vi "Read DIP Switches.vi"(8 "error in":errorcluster, 10 "Amount of Switches":i32=3, 11 "HBDeviceRef In":T1) -> (0 "error out":errorcluster, 1 "Boolean Array":bool[](array[boolean]), 2 "Index":dbl, 3 "HBDeviceRef Out":T1)   [LabVIEW 2016]
uses:
  <vilib>/Rock Robotics/WPI/SerialPort/WPI_SerialPortRef.ctl
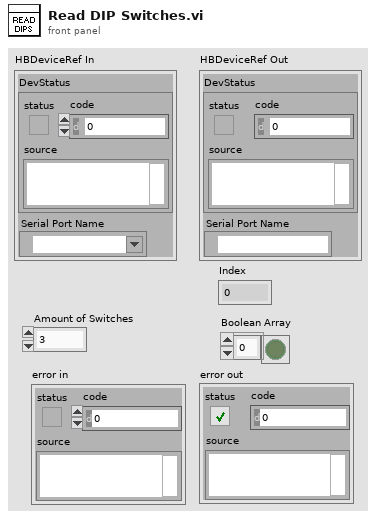
[diagram p1: front panel]
types:
  T1 = typedef "WPI_SerialPortRef.ctl" = cluster{"DevStatus":errorcluster, "Serial Port Name":refnum<visa-resource-name>}
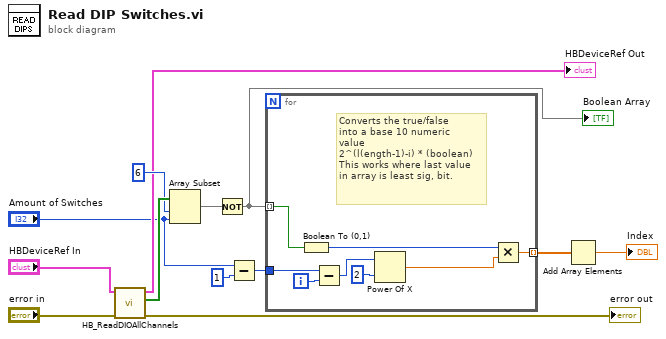
[diagram p0: block diagram]
diagram:
  n1 = call <vilib>:"HB_ReadDIOAllChannels.vi"("error in (no error)"="error in", "HBDeviceRef"="HBDeviceRef In") -> ("error out"=→"error out":errorcluster, "All Digital Input Vals"=w12:bool[], "HBDeviceRef"=→"HBDeviceRef Out":T1)  [unwired: 7 in]
  n2 = Array Subset(array=w12, index=6, length="Amount of Switches") -> (w10:bool[])
  n3 = Not(x=w10) -> (.not. x?=w9:bool[])
  "Boolean Array" <- w9
  n4 = Subtract(x="Amount of Switches", y=1) -> (x-y=w1:i32)
  n5 = for {
    tunnel: w9 -> [w16] mode=indexing
    tunnel: [w17] -> w13 mode=indexing
    tunnel: w1 -> [w14]
    i -> [w21]
    # "Converts the true/false\ninto a base 10 numeric\nvalue\n2^(l(ength-1)-i) * (boolean)\nThis works where last value \nin array is least sig, bit."
    n6 = Boolean To (0,1)(Boolean=w16) -> (0, 1=w15:i16)
    n7 = Subtract(x=w14, y=w21) -> (x-y=w19:i32)
    n8 = Power Of X(1:2, 2:w19) -> (0:w18:dbl)
    n9 = Multiply(x=w15, y=w18) -> (x*y=w17:dbl)
  }
  n10 = Add Array Elements(numeric array=w13) -> (sum=→"Index":dbl)
